vi "Main_v3.vi"() -> ()   [LabVIEW 2018]
uses:
  <vilib>/platform/TimedLoop/XDataNode/XDataNode.xnode
  <vilib>/Platform/TimedLoop/XDataNode/nitl_modes.ctl
  <vilib>/Platform/TimedLoop/XDataNode/XDNodeRunTimeDep.lvlib
  <vilib>/Platform/TimedLoop/XDataNode/wakeup.ctl
  <vilib>/Platform/TimedLoop/XDataNode/timing_clust.ctl
  Clusters/RoscoParams.ctl
  Clusters/SwapIn.ctl
  Clusters/SwapIndexes.ctl
  Clusters/FileDataChannel.ctl
  Clusters/SimulationConstants.ctl
  <vilib>/Utility/file.llb/Read Delimited Spreadsheet (DBL).vi
  <vilib>/Analysis/Matrix/Datatypes/RealMatrix.ctl
  <vilib>/Analysis/Matrix/NI_Matrix.lvlib
panel:
  out "Iteration Duration":i64
  out "Generator Speed (rad/s)":sgl(slide)=7.06858e-05 scale=-4.0..4.0
  in  "?":T1(tab)
  out "Generator Speed":sgl(graph)
  out "Torque Setpoint (kNm)":sgl(graph)
  out "Pitch Setpoint":sgl(graph)
  in  "To VS_ControlMode":T2(ring)
  in  "Edit DISCON":bool
  out "DISCON.IN Contents":string
  in  "From VS_ControlMode":T2(ring)
  out "avrSWAP":sgl[](array[numeric])
  out "Velocity":dbl
  out "Position":dbl
  out "Cp":dbl[][](array[numeric])
  out "Rotor Speed (rad/s)":sgl(slide)=7.06858e-05 scale=-4.0..4.0
  out "Torque Setpoint (kNm)":sgl(knob) scale=0.0..21586451.0
  out "Pitch Setpoint":sgl(knob) scale=0.0..1.5
  out "Power (kW)":sgl(slide) scale=-15000.0..15000.0 scale format="%.2f"
  in  "Init WindSpeed(m/s)":sgl=7.0
  in  "File path":path=path "/home/lvuser/rosco-tests"
  out "SimLoop Late?":bool
  out "FIFO Loop Late?":bool
  in  "Base filename":string="rosco-tests"
  out "Writing to cRIO?":bool
  in  "WriteData":bool
  in  "?":T3
  out "#RT FIFO":u32
  out "Call to Rosco Failed?":bool
  out "Rosco Return Message":string
  in  "?":bool
  out "time(s)":dbl
  out "RT Loop Late?":bool
  # "FOCAL Realtime Control (IEA 15MW)"
  # "SENSOR INPUTS"
  # "FILEWRITING SETTINGS"
  # "ERRORS"
  # "TURBINE SPECIFICATIONS"
  # "ROSCO OUTPUTS"
  # "RATED POWER: 15000000 W"
  # "RATED TORQUE: 19624046.66 Nm"
  # "RATED GEN SPEED: 0.79168 rad/s"
  # "ROSCO INPUTS"
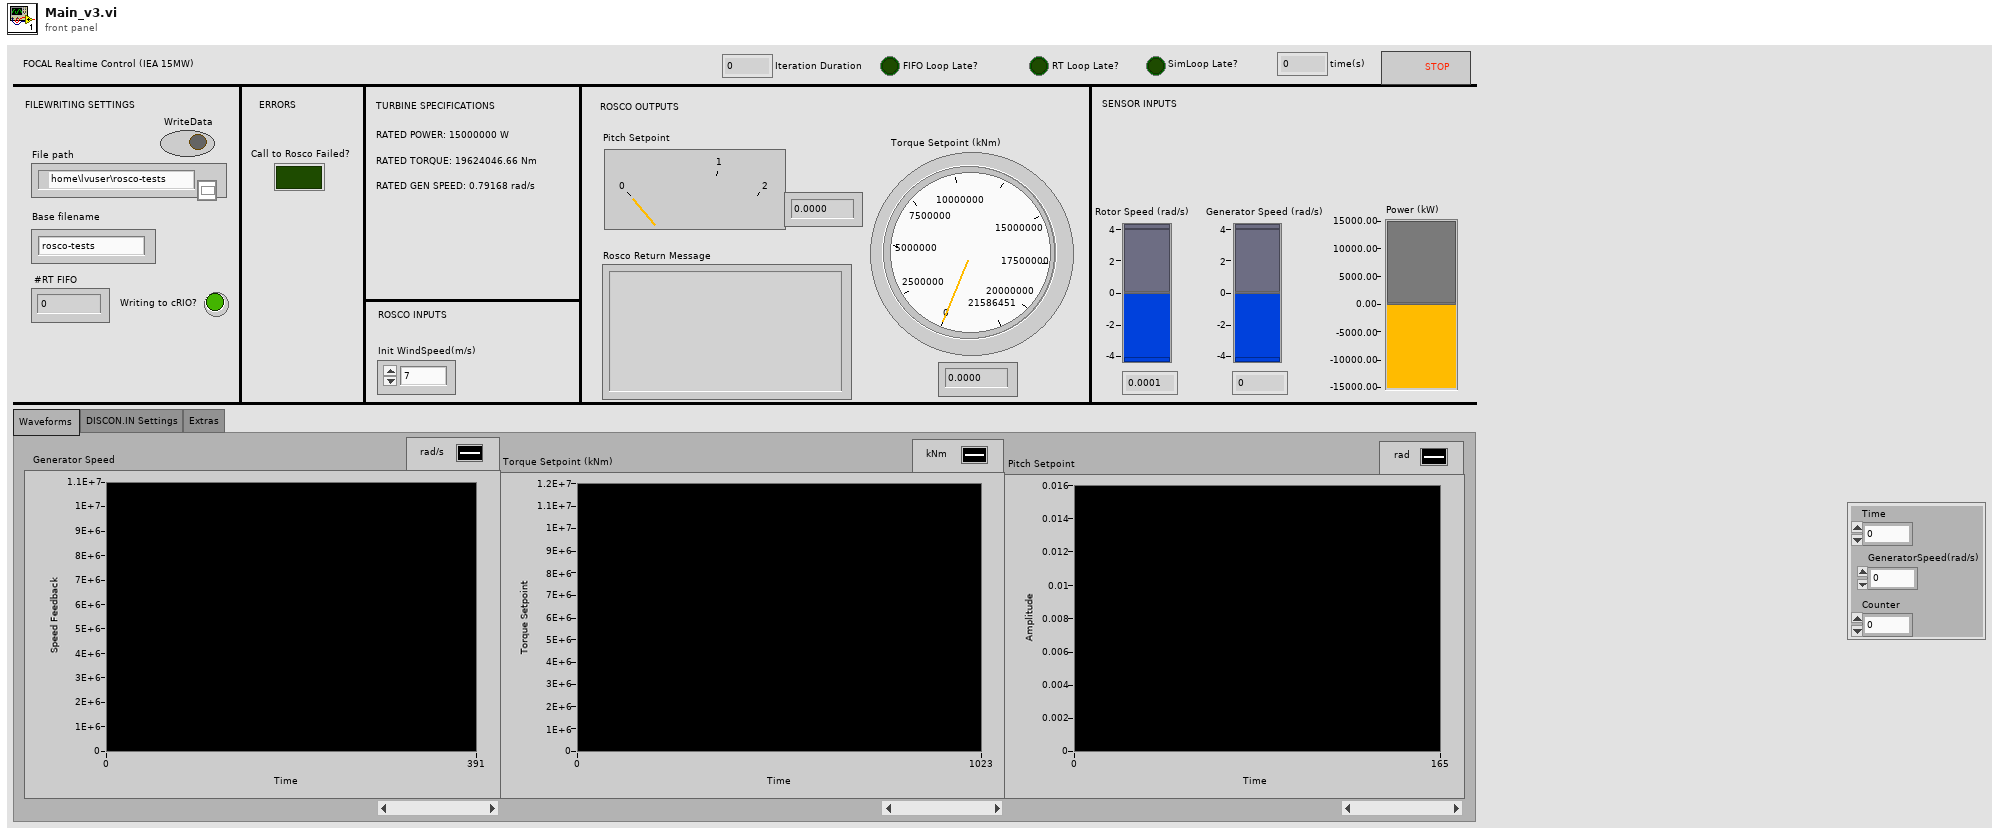
[diagram p1: front panel]
types:
  T1 = enum32{"Waveforms", "DISCON.IN Settings", "Extras"}
  T2 = enum16{"Constant Torque", "Constant Power", "PI Control"}
  T3 = typedef "FileDataChannel.ctl" = cluster{"GeneratorSpeed(rad/s)":sgl, "Counter":sgl, "Time":sgl}
  T4 = typedef "NI_Matrix.lvlib/RealMatrix.ctl" = dbl[][]
  T5 = typedef "SwapIndexes.ctl" = cluster{"iSTATUS":i32, "TIME":i32, "DT":i32, "BL_PITCH_1":i32, "VS_MECHGENPWR":i32, "GEN_SPEED":i32, "ROT_SPEED":i32, "GENTQMEAS":i32, "Y_M":i32, "HORWINDV":i32, "ROOTMOOP1":i32, "ROOTMOOP2":i32, "BL_PITCH_2":i32, "BL_PITCH_3":i32, "ROOTMOOP3":i32, "INFILE_SIZE":i32, "FA_ACC":i32, "NUM_BLADES":i32, " OUT BL_PITCH":i32, "OUT_ TORQUE":i32, "OUTFILE_SIZE ":i32, "AVCMSG_SIZE":i32, "AERODYN TQ":i32, "VS_GENPWR":i32}
  T6 = typedef "SwapIn.ctl" = cluster{"BladePitch(rad)":sgl, "RotorSpeed(rad/s)":sgl, "GeneratorSpeed(rad/s)":sgl, " GeneratorTorque(Nm)":sgl, " Generator Power(W) ":sgl, " WindSpeed(m/s)":sgl, "aviMSGLength":sgl, "InfileLength":sgl, "OutfileLength":sgl, "iStatus":sgl, "Time":sgl, "Dt":sgl, "NumberofBlades":sgl}
  T7 = typedef "RoscoParams.ctl" = cluster{"avrSWAP":sgl[], "aviFAIL":i32, "avcMSG":string, "ReturnValue":i32}
  T8 = typedef "XDNodeRunTimeDep.lvlib/timing_clust.ctl" = cluster{"Expected End [f-1]":u64, "Actual End [f-1]":u64, "Finished Late? [f-1]":bool, "Expected End [i-1]":u64, "Actual End [i-1]":u64, "Finished Late? [i-1]":bool, "Expected Start [i]":u64, "Actual Start [i]":u64, "Expected Start [f]":u64, "Actual Start [f]":u64, "Source Name":string, "Structure Name":string, "Period":i64, "Deadline":i64, "Offset":i64, "Start":i64, "Priority":i32, "Timeout":i32, "Mode":T9, "Wakeup Reason":T10, "Error":errorcluster, "Source Type":string, "Secondary Source Type":string, "Global End Time":u64, "Global Start Time":u64, "Frame Duration":u64, "Iteration Duration":u64, "Assigned CPU":i32, "I/O Scan Engine Mode":u32}
  T9 = typedef "XDNodeRunTimeDep.lvlib/nitl_modes.ctl" = enum32{"No Change", "Process missed periods, maintain original phase", "Discard missed periods, maintain original phase", "Process missed periods, ignore original phase", "Discard missed periods, ignore original phase"}
  T10 = typedef "XDNodeRunTimeDep.lvlib/wakeup.ctl" = enum32{"Normal", "Aborted", "Asynchronous wakeup", "Timing source error", "Timed loop error", "Timeout"}
  T11 = typedef "SimulationConstants.ctl" = cluster{"Ngear":sgl, "RotorInertia":sgl, "GeneratorEff":sgl, "RotorRadius":sgl, "Rho":sgl}
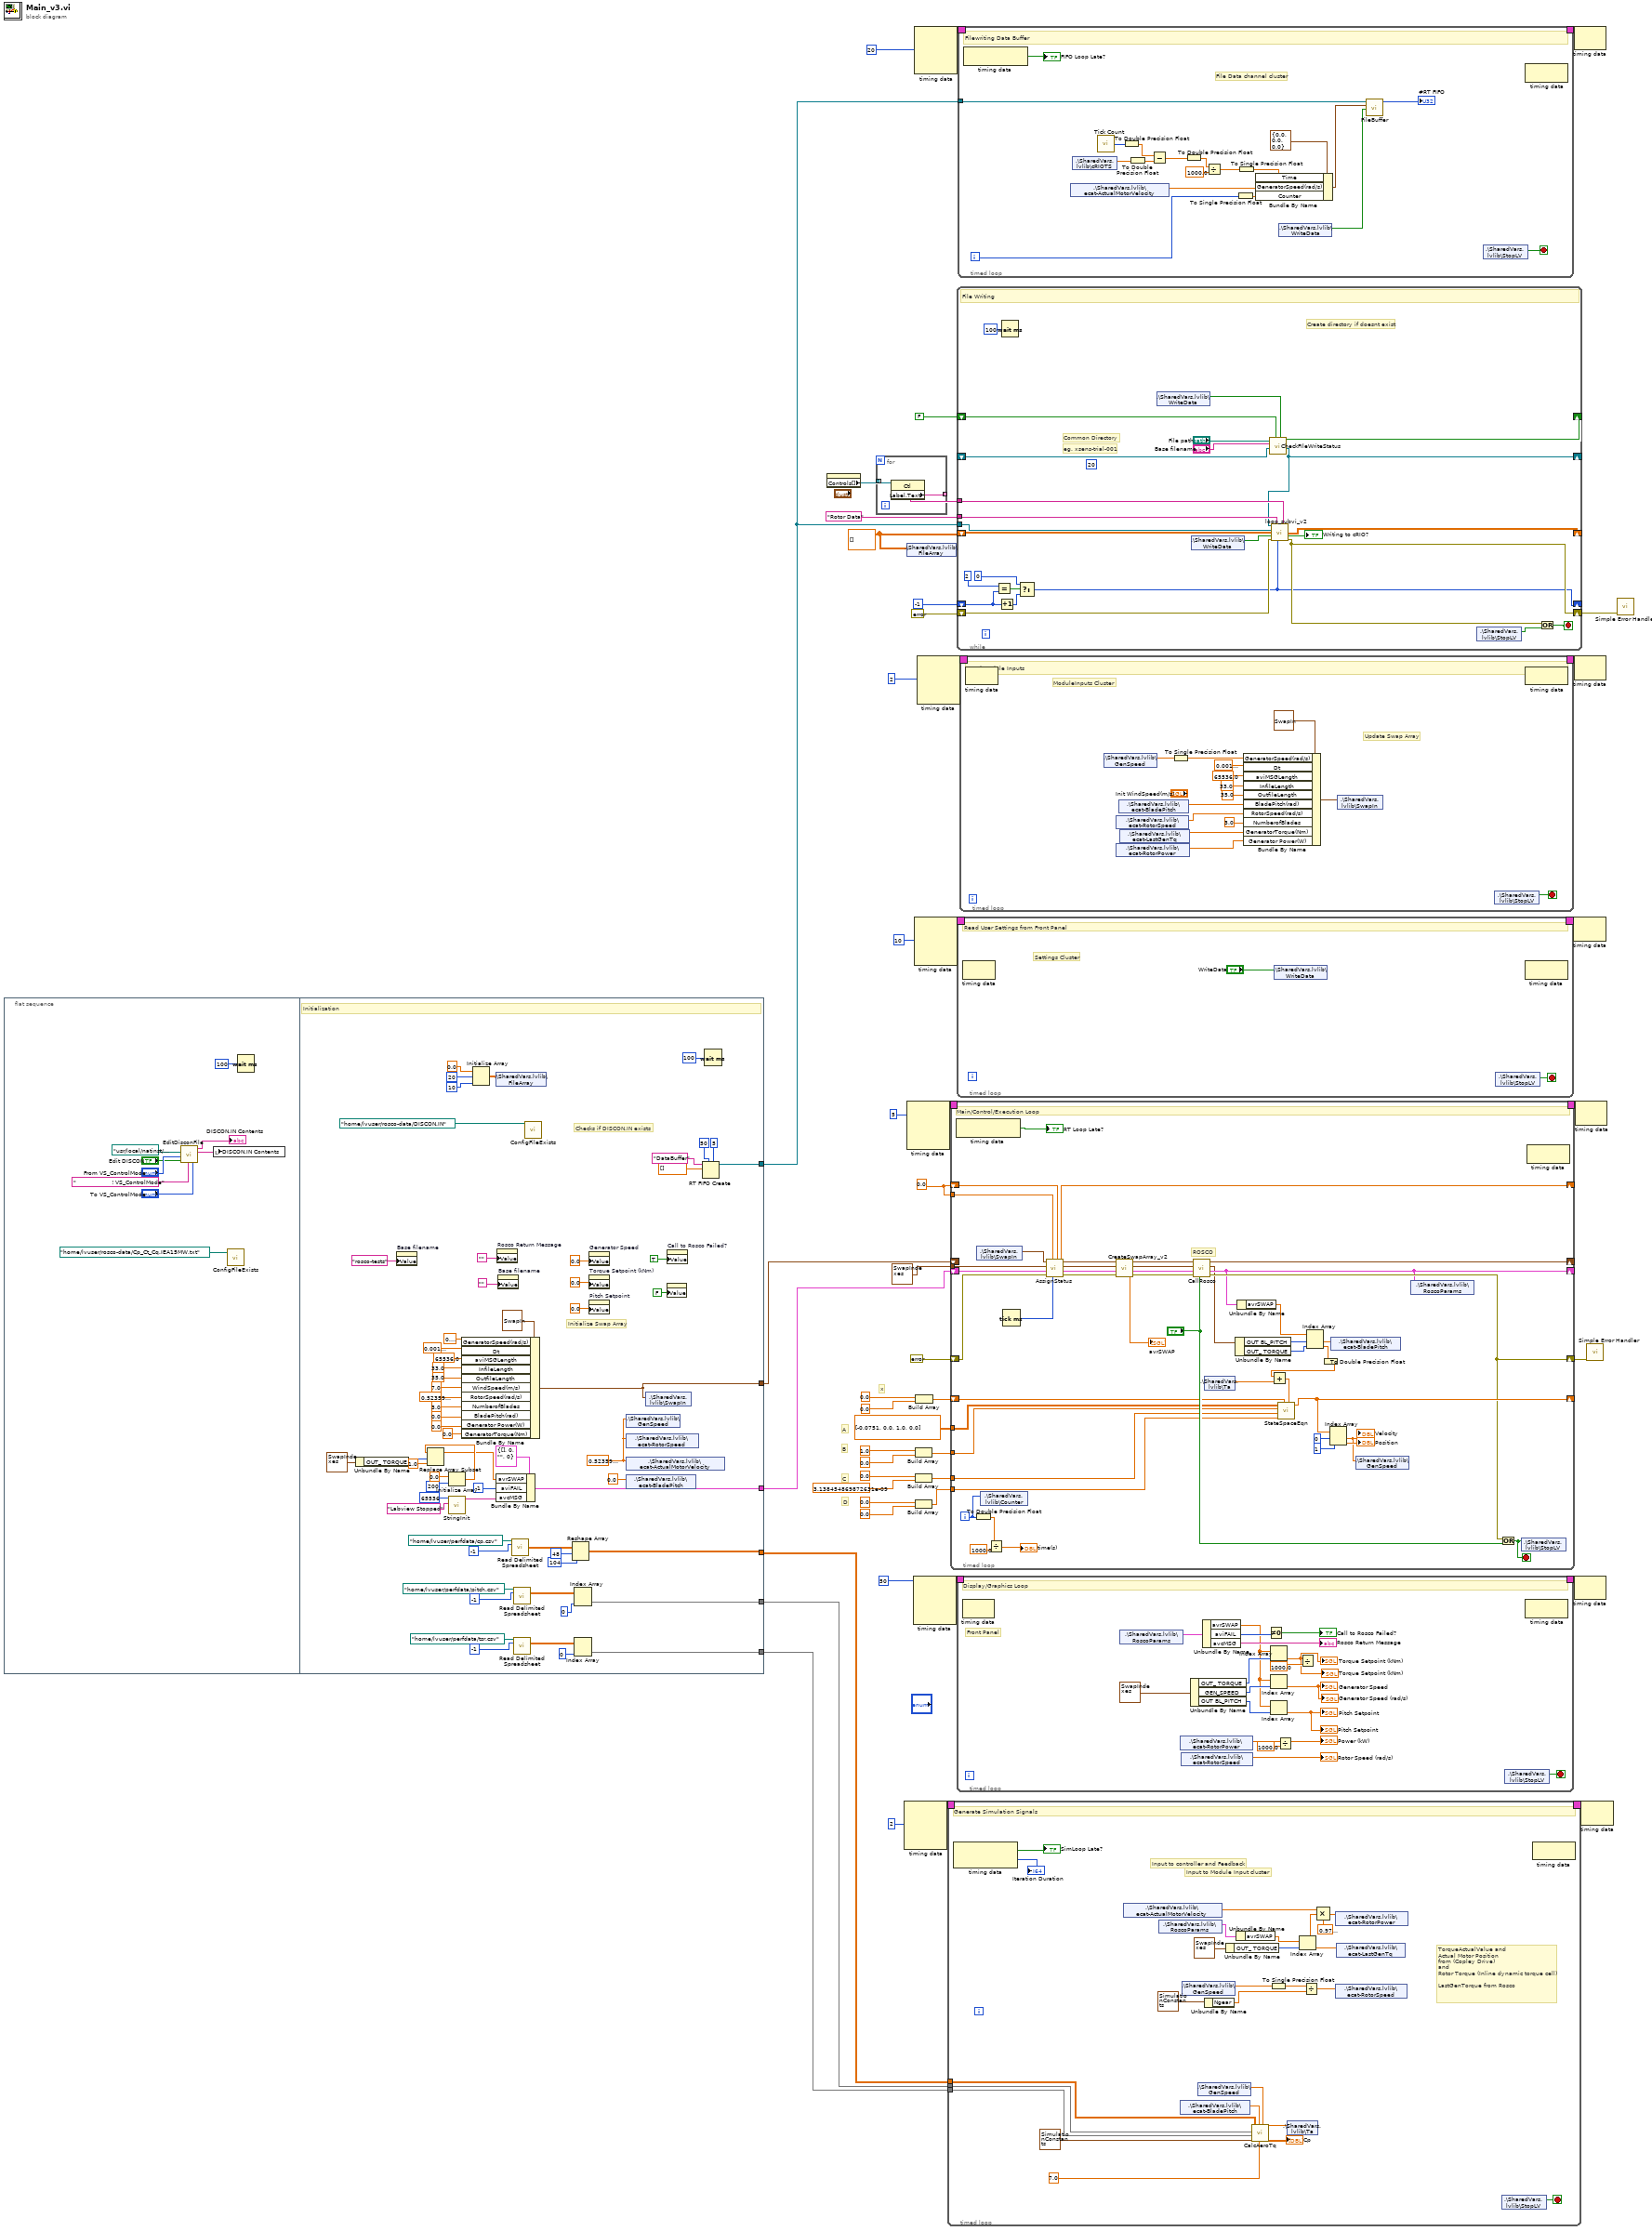
[diagram p0: block diagram]
diagram:
  w26 = dbl[][] [] ("File array 2")
  w33 = 0.0 ("y")
  (unwired) i64 20 ("Period")
  # "A"
  # "B"
  # "D"
  # "C"
  # "x"
  n1 = flat-sequence {
    tunnel: [w112] -> w27
    tunnel: [w86] -> w19
    tunnel: [w84] -> w5
    tunnel: [w73] -> w17
    tunnel: [w68] -> w16
    tunnel: [w67] -> w15
    frame #0 {
      n2 = call "EditDisconFile.vi"("To VS_ControlMode"="To VS_ControlMode", "Append"="                   ! VS_ControlMode", "Edit DISCON"="Edit DISCON", "From VS_ControlMode"="From VS_ControlMode", "path"=path "/usr/local/natinst/labview/DISCON.IN") -> ("result string"=w52:string, "data"=→"DISCON.IN Contents":string)  [unwired: 4 in]
      n3 = local write "DISCON.IN Contents"(w52) -> ()
      n4 = call "ConfigFileExists.vi"("path"=path "/home/lvuser/rosco-data/Cp_Ct_Cq.IEA15MW.txt") -> ()  [unwired: 11 in]
      n5 = Wait (ms)(milliseconds to wait=u32 100) -> ()  [unwired: 1 out]
    }
    frame #1 {
      w60 = sgl 0.5236 ("RotorSpeed(rad/s)")
      # "Initialize Swap Array"
      # "Checks if DISCON.IN exists"
      # "Initialization"
      n6 = Unbundle By Name(T5 {"iSTATUS"=0, "TIME"=1, "DT"=2, "BL_PITCH_1"=3, "VS_MECHGENPWR"=13, "GEN_SPEED"=19, "ROT_SPEED"=20, "GENTQMEAS"=22, "Y_M"=23, "HORWINDV"=26, "ROOTMOOP1"=29, "ROOTMOOP2"=30, "BL_PITCH_2"=32, "BL_PITCH_3"=33, "ROOTMOOP3"=31, "INFILE_SIZE"=49, "FA_ACC"=52, "NUM_BLADES"=60, " OUT BL_PITCH"=44, "OUT_ TORQUE"=46, "OUTFILE_SIZE "=50, "AVCMSG_SIZE"=48, "AERODYN TQ"=89, "VS_GENPWR"=14} ("Index In")) -> ("OUT_ TORQUE"=w64:i32)
      n7 = property on="Base filename" class="Str"("Value"="rosco-tests" ("Base filename")) -> ()  [unwired: 2 in, 2 out]
      n8 = Initialize Array(sgl 0.0 ("element"), 200 ("dimension size")) -> (w62:sgl[])
      n9 = Replace Array Subset(array=w62, new element=1.0 ("new element/subarray"), index=w64) -> (w61:sgl[])
      n10 = call "StringInit.vi"("accOUTNAME"="Labview Stopped", "dimension size"=65536) -> ("result string"=w116:string)  [unwired: 9 in]
      n11 = Bundle By Name(cluster=T6 {"BladePitch(rad)"=0.0, "RotorSpeed(rad/s)"=0.0, "GeneratorSpeed(rad/s)"=0.0, " GeneratorTorque(Nm)"=0.0, " Generator Power(W) "=0.0, " WindSpeed(m/s)"=0.0, "aviMSGLength"=0.0, "InfileLength"=0.0, "OutfileLength"=0.0, "iStatus"=0.0, "Time"=0.0, "Dt"=0.0, "NumberofBlades"=0.0}, "GeneratorSpeed(rad/s)"=sgl 0.3, "Dt"=sgl 0.001, "aviMSGLength"=sgl 65536.0 ("new element/subarray"), "InfileLength"=sgl 33.0 ("new element/subarray"), "OutfileLength"=sgl 35.0 ("new element/subarray"), "WindSpeed(m/s)"=sgl 7.0, "RotorSpeed(rad/s)"=sgl 0.5236, "NumberofBlades"=sgl 3.0, "BladePitch(rad)"=sgl 0.0, "Generator Power(W)"=sgl 0.0, "GeneratorTorque(Nm)"=sgl 0.0) -> (w84:T6)
      n12 = Initialize Array(0.0 ("element"), 20 ("dimension size"), 10 ("dimension size")) -> (w108:dbl[][])
      n13 = shared-variable ".\\SharedVars.lvlib\\FileArray"(w108) -> ()  [unwired: 1 in, 1 out]
      n14 = Bundle By Name(cluster=T7 {"avrSWAP"=[], "aviFAIL"=0, "avcMSG"="", "ReturnValue"=0}, "avrSWAP"=w61, "aviFAIL"=-1, "avcMSG"=w116) -> (w86:T7)
      n15 = property on="Rosco Return Message" class="Str"("Value"="") -> ()  [unwired: 2 in, 2 out]
      n16 = property on="Base filename" class="Str"("Value"="") -> ()  [unwired: 2 in, 2 out]
      n17 = call-poly <vilib>:"Read Delimited Spreadsheet.vi"("file path (dialog if empty)"=path "/home/lvuser/perfdata/cp.csv", "number of rows (all:-1)"=-1) -> ("all rows"=w76:dbl[][])  [unwired: 8 in, 5 out]
      n18 = call-poly <vilib>:"Read Delimited Spreadsheet.vi"("file path (dialog if empty)"=path "/home/lvuser/perfdata/pitch.csv", "number of rows (all:-1)"=-1) -> ("all rows"=w72:dbl[][])  [unwired: 8 in, 5 out]
      n19 = call-poly <vilib>:"Read Delimited Spreadsheet.vi"("file path (dialog if empty)"=path "/home/lvuser/perfdata/tsr.csv", "number of rows (all:-1)"=-1) -> ("all rows"=w78:dbl[][])  [unwired: 8 in, 5 out]
      n20 = call "ConfigFileExists.vi"("path"=path "/home/lvuser/rosco-data/DISCON.IN") -> ()  [unwired: 11 in]
      n21 = Reshape Array(w76, 48 ("dimension size"), 104 ("dimension size")) -> (w73:dbl[][])
      n22 = Index Array(array=w72, index (col)=0 ("disabled index (col)")) -> (element=w68:dbl[])  [unwired: 1 in]
      n23 = Index Array(array=w78, index (col)=0 ("disabled index (col)")) -> (element=w67:dbl[])  [unwired: 1 in]
      n24 = property on="Generator Speed" class="WFChart (strict)"("Value"=sgl 0.0 ("Generator Speed")) -> ()  [unwired: 2 in, 2 out]
      n25 = property on="Torque Setpoint (kNm)" class="WFChart (strict)"("Value"=sgl 0.0 ("Generator Speed")) -> ()  [unwired: 2 in, 2 out]
      n26 = property on="Pitch Setpoint" class="WFChart (strict)"("Value"=sgl 0.0 ("Generator Speed")) -> ()  [unwired: 2 in, 2 out]
      n27 = shared-variable ".\\SharedVars.lvlib\\GenSpeed"(w60) -> ()  [unwired: 1 in, 1 out]
      n28 = shared-variable ".\\SharedVars.lvlib\\ecat-RotorSpeed"(w60) -> ()  [unwired: 1 in, 1 out]
      n29 = shared-variable ".\\SharedVars.lvlib\\ecat-ActualMotorVelocity"(w60) -> ()  [unwired: 1 in, 1 out]
      n30 = shared-variable ".\\SharedVars.lvlib\\ecat-BladePitch"(sgl 0.0 ("ecat-BladePitch")) -> ()  [unwired: 1 in, 1 out]
      n31 = shared-variable ".\\SharedVars.lvlib\\SwapIn"(w84) -> ()  [unwired: 1 in, 1 out]
      n32 = property class="Bool (strict)"("Value"=FALSE) -> ()  [unwired: 2 in, 2 out]
      n33 = property on="Call to Rosco Failed?" class="Bool (strict)"("Value"=TRUE ("Call to Rosco Failed?")) -> ()  [unwired: 2 in, 2 out]
      n34 = RT FIFO Create(0:"DataBuffer" ("name (unnamed)"), 1:dbl[] [] ("appended array"), 4:u32 50, 6:u32 5) -> (8:w112:refnum<k33>)  [unwired: 4 in, 2 out]
      n35 = Wait (ms)(milliseconds to wait=u32 100) -> ()  [unwired: 1 out]
    }
  }
  n36 = property class="Clust (strict)"() -> ("Controls[]"=w30:refnum<vi>[])  [unwired: 2 in, 2 out]
  n37 = for {
    tunnel: w30 -> [w123] mode=indexing
    tunnel: [w122] -> w29 mode=indexing
    n38 = property class="Ctl"(reference=w123) -> ("Label.Text"=w122:string)  [unwired: 1 in, 2 out]
  }
  n39 = node-c288(i64 2 ("Period")) -> (w41:T8)  [unwired: 3 in]
  n40 = shared-variable ".\\SharedVars.lvlib\\FileArray"(w26) -> ()  [unwired: 1 in, 1 out]
  n41 = node-c288(i64 5 ("Period")) -> (w39:T8)  [unwired: 3 in]
  n42 = node-c288(i64 50 ("Period")) -> (w43:T8)  [unwired: 3 in]
  n43 = node-c288(i64 10 ("Period")) -> (w45:T8)  [unwired: 3 in]
  n44 = node-c288(i64 20 ("Period")) -> (w49:T8)  [unwired: 3 in]
  n45 = Build Array(1.0 ("element"), 0.0 ("element")) -> (w3:dbl[])
  n46 = Build Array(0.0 ("element"), 3.138454869872631e-09 ("element")) -> (w2:dbl[])
  n47 = Build Array(0.0 ("element"), 0.0 ("element")) -> (w1:dbl[])
  n48 = Build Array(0.0 ("element"), 0.0 ("element")) -> (w10:dbl[])
  n49 = node-c288(i64 2 ("Period")) -> (w47:T8)  [unwired: 3 in]
  n50 = timed-loop {
    timing: w41 -> [_]
    timing-out: [_] -> w40
    tunnel: w17 -> [w130]
    tunnel: w16 -> [w129]
    tunnel: w15 -> [w128]
    stop <- w148 stop-if-true
    # "TorqueActualValue and \nActual Motor Position \nfrom (Copley Drive)\nand\nRotor Torque (Inline dynamic torque cell)\n\nLastGenTorque from Rosco"
    # "Input to Module Input cluster"
    # "Input to controller and Feedback"
    # "Generate Simulation Signals"
    n51 = node-c288() -> (→"SimLoop Late?":bool, →"Iteration Duration":i64)  [unwired: 1 in]
    n52 = shared-variable ".\\SharedVars.lvlib\\ecat-ActualMotorVelocity"() -> (w142:sgl)  [unwired: 1 in, 1 out]
    n53 = shared-variable ".\\SharedVars.lvlib\\RoscoParams"() -> (w141:T7)  [unwired: 1 in, 1 out]
    n54 = shared-variable ".\\SharedVars.lvlib\\ecat-BladePitch"() -> (w132:sgl)  [unwired: 1 in, 1 out]
    n55 = shared-variable ".\\SharedVars.lvlib\\GenSpeed"() -> (w136:dbl)  [unwired: 1 in, 1 out]
    n56 = shared-variable ".\\SharedVars.lvlib\\GenSpeed"() -> (w131:dbl)  [unwired: 1 in, 1 out]
    n57 = Unbundle By Name(T11 {"Ngear"=1.0, "RotorInertia"=318628130.0, "GeneratorEff"=0.97, "RotorRadius"=0.97, "Rho"=0.97} ("SimulationConst")) -> ("Ngear"=w138:sgl)
    n58 = Unbundle By Name(T5 {"iSTATUS"=0, "TIME"=1, "DT"=2, "BL_PITCH_1"=3, "VS_MECHGENPWR"=13, "GEN_SPEED"=19, "ROT_SPEED"=20, "GENTQMEAS"=22, "Y_M"=23, "HORWINDV"=26, "ROOTMOOP1"=29, "ROOTMOOP2"=30, "BL_PITCH_2"=32, "BL_PITCH_3"=33, "ROOTMOOP3"=31, "INFILE_SIZE"=49, "FA_ACC"=52, "NUM_BLADES"=60, " OUT BL_PITCH"=44, "OUT_ TORQUE"=46, "OUTFILE_SIZE "=50, "AVCMSG_SIZE"=48, "AERODYN TQ"=89, "VS_GENPWR"=14} ("Index In")) -> ("OUT_ TORQUE"=w143:i32)
    n59 = Unbundle By Name(w141) -> ("avrSWAP"=w144:sgl[])
    n60 = call "CalcAeroTq.vi"("GenSpeed"=w131, "WindSpeed"=sgl 7.0, "Xi"=w132, "SimulationConst"=T11 {"Ngear"=1.0, "RotorInertia"=318628130.0, "GeneratorEff"=0.97, "RotorRadius"=0.97, "Rho"=0.97}, "tsr(Y)"=w128, "pitch (X)"=w129, "Cp(Z)"=w130) -> ("Cp"=→"Cp":dbl[][], "Ta"=w124:dbl)  [unwired: 3 in]
    n61 = To Single Precision Float(number=w136) -> (single precision float=w135:sgl)
    n62 = shared-variable ".\\SharedVars.lvlib\\Ta"(w124) -> ()  [unwired: 1 in, 1 out]
    n63 = Index Array(array=w144, index=w143) -> (element=w147:sgl)
    n64 = Divide(x=w135, y=w138) -> (x/y=w137:sgl)
    n65 = Compound Arithmetic op=MULTIPLY(w142, w147, sgl 0.97 ("value")) -> (w145:sgl)
    n66 = shared-variable ".\\SharedVars.lvlib\\ecat-RotorPower"(w145) -> ()  [unwired: 1 in, 1 out]
    n67 = shared-variable ".\\SharedVars.lvlib\\ecat-RotorSpeed"(w137) -> ()  [unwired: 1 in, 1 out]
    n68 = shared-variable ".\\SharedVars.lvlib\\ecat-LastGenTq"(w147) -> ()  [unwired: 1 in, 1 out]
    n69 = shared-variable ".\\SharedVars.lvlib\\StopLV"() -> (w148:bool)  [unwired: 1 in, 1 out]
    n70 = node-c288() -> ()  [unwired: 1 in, 1 out]
  }
  n71 = timed-loop {
    timing: w39 -> [_]
    timing-out: [_] -> w38
    shift-right: [w190] -> _
    shift-left: w33 -> [w192]
    tunnel: w33 -> [w191]
    tunnel: T5 {"iSTATUS"=0, "TIME"=1, "DT"=2, "BL_PITCH_1"=3, "VS_MECHGENPWR"=13, "GEN_SPEED"=19, "ROT_SPEED"=20, "GENTQMEAS"=22, "Y_M"=23, "HORWINDV"=26, "ROOTMOOP1"=29, "ROOTMOOP2"=30, "BL_PITCH_2"=32, "BL_PITCH_3"=33, "ROOTMOOP3"=31, "INFILE_SIZE"=49, "FA_ACC"=52, "NUM_BLADES"=60, " OUT BL_PITCH"=44, "OUT_ TORQUE"=46, "OUTFILE_SIZE "=50, "AVCMSG_SIZE"=48, "AERODYN TQ"=89, "VS_GENPWR"=14} ("Index In") -> [w194]
    shift-right: [w155] -> _
    shift-left: w19 -> [w193]
    shift-right: [w186] -> _
    shift-left: w5 -> [_]
    shift-right: [w156] -> w20
    shift-left: errorcluster {"status"=FALSE, "code"=0, "source"=""} ("error out") -> [w189]
    shift-right: [w169] -> _
    shift-left: w10 -> [w174]
    tunnel: T4 [[-0.0751, 0.0], [1.0, 0.0]] ("A") -> [w173]
    tunnel: w3 -> [w172]
    tunnel: w2 -> [w171]
    tunnel: w1 -> [w170]
    i -> [w185]
    stop <- w187 stop-if-true
    # "ROSCO"
    # "Main/Control/Execution Loop"
    n72 = node-c288() -> (→"RT Loop Late?":bool)  [unwired: 1 in]
    n73 = To Double Precision Float(number=w185) -> (double precision float=w197:dbl)
    n74 = shared-variable ".\\SharedVars.lvlib\\SwapIn"() -> (w162:T6)  [unwired: 1 in, 1 out]
    n75 = shared-variable ".\\SharedVars.lvlib\\Counter"(w185) -> ()  [unwired: 1 in, 1 out]
    n76 = Divide(x=w197, y=1000.0) -> (x/y=→"time(s)":dbl)
    n77 = Tick Count (ms)() -> (millisecond timer value=w184:u32)
    n78 = call "AssignStatus.vi"("LoopCount"=w192, "Time"=w184, "Init Val"=w191, "error in (no error)"=w189, "ROSCO Params"=w193, 10:w194, "SwapIn"=w162) -> ("error out"=w180:errorcluster, "ROSCO Params 2"=w181:T7, 2:w182:T5, "SwapIn"=w183:T6, "Count+1"=w190:dbl)
    n79 = call "CreateSwapArray_v2.vi"("error in (no error)"=w180, "ROSCO Params"=w181, "Index In"=w182, "SwapIn"=w183) -> ("error out"=w176:errorcluster, "ROSCO Params Out"=w177:T7, "Index Out"=w178:T5, "SwapIn Out"=w179:T6, "avrSWAP"=→"avrSWAP":sgl[])  [unwired: 3 in]
    n80 = call "CallRosco.vi"("StopLV"="?", "error in (no error)"=w176, "ROSCO Params in"=w177, "Index In"=w178, "SwapIn"=w179) -> ("error out"=w156:errorcluster, "ROSCO Params out"=w155:T7, "IndexOut"=w154:T5, "SwapOut"=w186:T6)  [unwired: 3 in]
    n81 = shared-variable ".\\SharedVars.lvlib\\Ta"() -> (w157:dbl)  [unwired: 1 in, 1 out]
    n82 = Unbundle By Name(w154) -> ("OUT BL_PITCH"=w164:i32, "OUT_ TORQUE"=w161:i32)
    n83 = Unbundle By Name(w155) -> ("avrSWAP"=w165:sgl[])
    n84 = Index Array(array=w165, index #1=w164, index #2=w161) -> (element #1=w159:sgl, element #2=w160:sgl)
    n85 = To Double Precision Float(number=w160) -> (double precision float=w158:dbl)
    n86 = Add(x=w158, y=w157) -> (x+y=w153:dbl)
    n87 = call "StateSpaceEqn.vi"("u"=w153, "x"=w174, "D"=w170, "C"=w171, "B"=w172, "A"=w173) -> ("x(t+1)"=w169:dbl[])  [unwired: 4 in, 1 out]
    n88 = Index Array(array=w169, index #1=0 ("index"), index #2=1 ("index")) -> (element #1=w163:dbl, element #2=→"Position":dbl)
    "Velocity" <- w163
    n89 = shared-variable ".\\SharedVars.lvlib\\ecat-BladePitch"(w159) -> ()  [unwired: 1 in, 1 out]
    n90 = shared-variable ".\\SharedVars.lvlib\\GenSpeed"(w163) -> ()  [unwired: 1 in, 1 out]
    n91 = shared-variable ".\\SharedVars.lvlib\\RoscoParams"(w155) -> ()  [unwired: 1 in, 1 out]
    n92 = Or(x=w156, y="?") -> (x .or. y?=w187:bool)
    n93 = shared-variable ".\\SharedVars.lvlib\\StopLV"(w187) -> ()  [unwired: 1 in, 1 out]
    n94 = node-c288() -> ()  [unwired: 1 in, 1 out]
  }
  n95 = timed-loop {
    timing: w43 -> [_]
    timing-out: [_] -> w42
    stop <- w219 stop-if-true
    # "Front Panel"
    # "Display/Graphics Loop"
    n96 = node-c288() -> ()  [unwired: 1 in, 1 out]
    n97 = shared-variable ".\\SharedVars.lvlib\\RoscoParams"() -> (w218:T7)  [unwired: 1 in, 1 out]
    n98 = shared-variable ".\\SharedVars.lvlib\\ecat-RotorPower"() -> (w208:sgl)  [unwired: 1 in, 1 out]
    n99 = shared-variable ".\\SharedVars.lvlib\\ecat-RotorSpeed"() -> (→"Rotor Speed (rad/s)":sgl)  [unwired: 1 in, 1 out]
    n100 = Unbundle By Name(T5 {"iSTATUS"=0, "TIME"=1, "DT"=2, "BL_PITCH_1"=3, "VS_MECHGENPWR"=13, "GEN_SPEED"=19, "ROT_SPEED"=20, "GENTQMEAS"=22, "Y_M"=23, "HORWINDV"=26, "ROOTMOOP1"=29, "ROOTMOOP2"=30, "BL_PITCH_2"=32, "BL_PITCH_3"=33, "ROOTMOOP3"=31, "INFILE_SIZE"=49, "FA_ACC"=52, "NUM_BLADES"=60, " OUT BL_PITCH"=44, "OUT_ TORQUE"=46, "OUTFILE_SIZE "=49, "AVCMSG_SIZE"=49, "AERODYN TQ"=46, "VS_GENPWR"=13}) -> ("OUT_ TORQUE"=w216:i32, "GEN_SPEED"=w215:i32, "OUT BL_PITCH"=w210:i32)
    n101 = Unbundle By Name(w218) -> ("avrSWAP"=w211:sgl[], "aviFAIL"=w213:i32, "avcMSG"=→"Rosco Return Message":string)
    n102 = Not Equal To 0?(x=w213) -> (x != 0?=→"Call to Rosco Failed?":bool)
    n103 = Index Array(array=w211, index=w216) -> (element=w202:sgl)
    "Torque Setpoint (kNm)" <- w202
    "Torque Setpoint (kNm)" <- w202
    n104 = Index Array(array=w211, index=w215) -> (element=→"Generator Speed" →"Generator Speed (rad/s)":sgl)
    n105 = Index Array(array=w211, index=w210) -> (element=→"Pitch Setpoint" →"Pitch Setpoint":sgl)
    n106 = Divide(x=w208, y=sgl 1000.0) -> (x/y=→"Power (kW)":sgl)
    n107 = Divide(x=w202, y=sgl 1000.0) -> ()  [unwired: 1 out]
    n108 = shared-variable ".\\SharedVars.lvlib\\StopLV"() -> (w219:bool)  [unwired: 1 in, 1 out]
    n109 = node-c288() -> ()  [unwired: 1 in, 1 out]
  }
  n110 = while {
    shift-right: [w222] -> _
    shift-left: _ -> [w223]
    shift-right: [w230] -> _
    shift-left: FALSE -> [w231]
    shift-right: [w243] -> w22
    shift-left: errorcluster {"status"=FALSE, "code"=0, "source"=""} ("error out") -> [w242]
    tunnel: "Rotor Data" -> [w225]
    tunnel: w29 -> [w226]
    tunnel: w27 -> [w227]
    shift-right: [w239] -> _
    shift-left: -1 -> [w241]
    shift-right: [w234] -> _
    shift-left: w26 -> [w240]
    stop <- w245 stop-if-true
    # "eg. xsens-trial-001"
    # "Create directory if doesnt exist"
    # "Common Directory"
    # "File Writing"
    n111 = Equal?(x=2 ("t"), y=w241) -> (x = y?=w236:bool)
    n112 = Increment(x=w241) -> (x+1=w235:i32)
    n113 = Wait (ms)(milliseconds to wait=u32 100) -> ()  [unwired: 1 out]
    n114 = Select(t=0, s=w236, f=w235) -> (s? t:f=w239:i32)
    n115 = shared-variable ".\\SharedVars.lvlib\\WriteData"() -> (w232:bool)  [unwired: 1 in, 1 out]
    n116 = shared-variable ".\\SharedVars.lvlib\\WriteData"() -> (w228:bool)  [unwired: 1 in, 1 out]
    n117 = call "CheckFIleWriteStatus.vi"("WriteDataButtonVal"=w232, "WritePrevVal"=w231, "Refnum in"=w223, "Base filename"="Base filename", "File path"="File path") -> ("Refnum out"=w222:refnum<k34>, "WriteCurrentVal"=w230:bool)  [unwired: 5 in]
    n118 = call "loop_subvi_v2.vi"("Refnum in"=w222, "Group Name"=w225, "Channel Names"=w226, "rt fifo"=w227, "File array"=w240, "Write?"=w228, "error in (no error)"=w242, "index"=w239) -> ("File array 2"=w234:dbl[][], "Writing to file"=→"Writing to cRIO?":bool, "error out"=w243:errorcluster)  [unwired: 4 in, 1 out]
    n119 = shared-variable ".\\SharedVars.lvlib\\StopLV"() -> (w246:bool)  [unwired: 1 in, 1 out]
    n120 = Or(x=w243, y=w246) -> (x .or. y?=w245:bool)
  }
  n121 = timed-loop {
    timing: w45 -> [_]
    timing-out: [_] -> w44
    stop <- w248 stop-if-true
    # "Settings Cluster"
    # "Read User Settings from Front Panel"
    n122 = node-c288() -> ()  [unwired: 1 in, 1 out]
    n123 = shared-variable ".\\SharedVars.lvlib\\WriteData"("WriteData") -> ()  [unwired: 1 in, 1 out]
    n124 = shared-variable ".\\SharedVars.lvlib\\StopLV"() -> (w248:bool)  [unwired: 1 in, 1 out]
    n125 = node-c288() -> ()  [unwired: 1 in, 1 out]
  }
  n126 = timed-loop {
    timing: w49 -> [_]
    timing-out: [_] -> w48
    tunnel: w27 -> [w257]
    i -> [w252]
    stop <- w269 stop-if-true
    # "File Data channel cluster"
    # "Filewriting Data Buffer"
    n127 = node-c288() -> (→"FIFO Loop Late?":bool)  [unwired: 1 in]
    n128 = shared-variable ".\\SharedVars.lvlib\\ecat-ActualMotorVelocity"() -> (w262:sgl)  [unwired: 1 in, 1 out]
    n129 = shared-variable ".\\SharedVars.lvlib\\cRIOTS"() -> (w264:dbl)  [unwired: 1 in, 1 out]
    n130 = call "Tick Count"() -> ("Tick Count(mSec)"=w265:u32)
    n131 = To Double Precision Float(number=w265) -> (double precision float=w254:dbl)
    n132 = To Double Precision Float(number=w264) -> (double precision float=w263:dbl)
    n133 = Subtract(x=w254, y=w263) -> (x-y=w266:dbl)
    n134 = To Double Precision Float(number=w266) -> (double precision float=w268:dbl)
    n135 = Divide(x=w268, y=1000.0) -> (x/y=w253:dbl)
    n136 = To Single Precision Float(number=w252) -> (single precision float=w255:sgl)
    n137 = To Single Precision Float(number=w253) -> (single precision float=w261:sgl)
    n138 = Bundle By Name(cluster=T3 {"GeneratorSpeed(rad/s)"=0.0, "Counter"=0.0, "Time"=0.0} ("SwapIn"), "Time"=w261, "GeneratorSpeed(rad/s)"=w262, "Counter"=w255) -> (w259:T3)
    n139 = shared-variable ".\\SharedVars.lvlib\\WriteData"() -> (w258:bool)  [unwired: 1 in, 1 out]
    n140 = call "FileBuffer.vi"("Boolean"=w258, "FileDataChannel"=w259, "Refnum in"=w257) -> ("# elements"=→"#RT FIFO":u32)  [unwired: 8 in]
    n141 = shared-variable ".\\SharedVars.lvlib\\StopLV"() -> (w269:bool)  [unwired: 1 in, 1 out]
    n142 = node-c288() -> ()  [unwired: 1 in, 1 out]
  }
  n143 = timed-loop {
    timing: w47 -> [_]
    timing-out: [_] -> w46
    stop <- w286 stop-if-true
    # "Update Swap Array"
    # "ModuleInputs Cluster"
    # "Read Module Inputs"
    n144 = node-c288() -> ()  [unwired: 1 in, 1 out]
    n145 = shared-variable ".\\SharedVars.lvlib\\GenSpeed"() -> (w279:dbl)  [unwired: 1 in, 1 out]
    n146 = shared-variable ".\\SharedVars.lvlib\\ecat-RotorSpeed"() -> (w276:sgl)  [unwired: 1 in, 1 out]
    n147 = shared-variable ".\\SharedVars.lvlib\\ecat-RotorPower"() -> (w273:sgl)  [unwired: 1 in, 1 out]
    n148 = shared-variable ".\\SharedVars.lvlib\\ecat-BladePitch"() -> (w277:sgl)  [unwired: 1 in, 1 out]
    n149 = shared-variable ".\\SharedVars.lvlib\\ecat-LastGenTq"() -> (w274:sgl)  [unwired: 1 in, 1 out]
    n150 = To Single Precision Float(number=w279) -> (single precision float=w278:sgl)
    n151 = Bundle By Name(cluster=T6 {"BladePitch(rad)"=0.0, "RotorSpeed(rad/s)"=0.0, "GeneratorSpeed(rad/s)"=0.0, " GeneratorTorque(Nm)"=0.0, " Generator Power(W) "=0.0, " WindSpeed(m/s)"=0.0, "aviMSGLength"=0.0, "InfileLength"=0.0, "OutfileLength"=0.0, "iStatus"=0.0, "Time"=0.0, "Dt"=0.0, "NumberofBlades"=0.0}, "GeneratorSpeed(rad/s)"=w278, "Dt"=sgl 0.001, "aviMSGLength"=sgl 65536.0 ("new element/subarray"), "InfileLength"=sgl 33.0 ("new element/subarray"), "OutfileLength"=sgl 35.0 ("new element/subarray"), "BladePitch(rad)"=w277, "RotorSpeed(rad/s)"=w276, "NumberofBlades"=sgl 3.0, "GeneratorTorque(Nm)"=w274, "Generator Power(W)"=w273) -> (w285:T6)
    n152 = shared-variable ".\\SharedVars.lvlib\\SwapIn"(w285) -> ()  [unwired: 1 in, 1 out]
    n153 = shared-variable ".\\SharedVars.lvlib\\StopLV"() -> (w286:bool)  [unwired: 1 in, 1 out]
    n154 = node-c288() -> ()  [unwired: 1 in, 1 out]
  }
  n155 = node-c288(w44) -> ()  [unwired: 1 out]
  n156 = node-c288(w48) -> ()  [unwired: 1 out]
  n157 = node-c288(w46) -> ()  [unwired: 1 out]
  n158 = node-c288(w42) -> ()  [unwired: 1 out]
  n159 = node-c288(w38) -> ()  [unwired: 1 out]
  n160 = node-c288(w40) -> ()  [unwired: 1 out]
  n161 = call <vilib>:"Simple Error Handler.vi"("error in (no error)"=w20) -> ()  [unwired: 4 in, 5 out]
  n162 = call <vilib>:"Simple Error Handler.vi"("error in (no error)"=w22) -> ()  [unwired: 4 in, 5 out]
